vi "Create.vi"(5 "JUnit for Azure Pipelines in":refnum<class "JUnit for Azure Pipelines.lvclass">, 8 "error in (no error)":errorcluster, 11 "Path":path) -> (0 "error out":errorcluster, 3 "JUnit for Azure Pipelines":refnum<class "JUnit for Azure Pipelines.lvclass">)   [LabVIEW 2013, in "JUnit for Azure Pipelines.lvclass"]
uses:
  JUnit for Azure Pipelines.lvclass
  <vilib>/addons/_JKI Toolkits/Caraya/classes/MsgSerializer.XML/MsgSerializer.XML.lvclass
  JUnit for Azure Pipelines.lvclass/JUnit for Azure Pipelines.ctl
  <vilib>/addons/_JKI Toolkits/Caraya/classes/Test Report/Test Report.lvclass/Test Report.ctl
  <vilib>/addons/_JKI Toolkits/Caraya/classes/Test Report/Test Report.lvclass
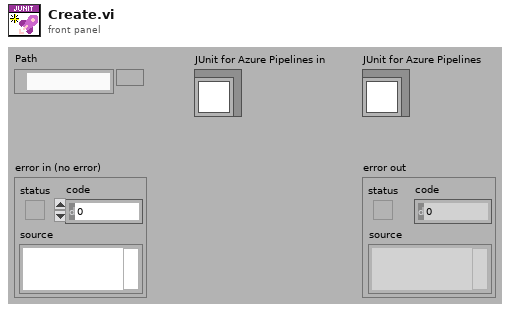
[diagram p1: front panel]
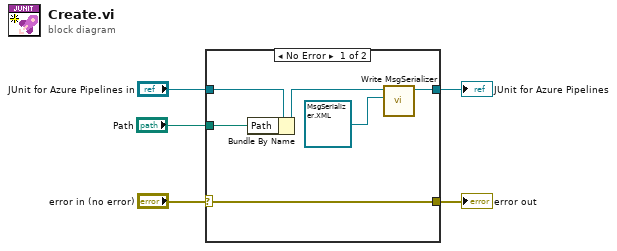
[diagram p0: block diagram]
diagram:
  n1 = case shown="No Error" "error in (no error)" {
    selector: "error in (no error)" -> [w11 w13]
    tunnel: [w11 w13] -> w4
    tunnel: [w6 w12] -> w2
    tunnel: "JUnit for Azure Pipelines in" -> [w10 w12]
    tunnel: "Path" -> [w9 _]
    frame No Error {
      n2 = Bundle By Name(cluster=w10, "Path"=w9) -> (w7:refnum<class "JUnit for Azure Pipelines.lvclass">)
      n3 = call <vilib>:"Write MsgSerializer.vi"("MsgSerializer"=refnum<class "MsgSerializer.XML.lvclass"> refnum ("Caraya.lvlib:MsgSerializer.XMLProperty.lvclass"), "Test Report in"=w7) -> ("Test Report out"=w6:refnum<class "JUnit for Azure Pipelines.lvclass">)  [unwired: 9 in]
    }
    frame Error {
    }
  }
  "error out" <- w4
  "JUnit for Azure Pipelines" <- w2
